vi "Select Trans.vi"(8 "error in (no error)":errorcluster) -> (0 "error out":errorcluster, 3 "Amplifier Type 2":T1)   [LabVIEW 2015]
uses:
  controls/OpAmp Amplifiers.ctl
  controls/AmplifierTypes.ctl
panel:
  in  "Cancel Button":bool
  in  "Amplifier Type":T1 caption="Trans Type"
  in  "Opamp Type":T2 caption="OpAmp"
  in  "EC":bool
  in  "CC":bool
  in  "BC":bool
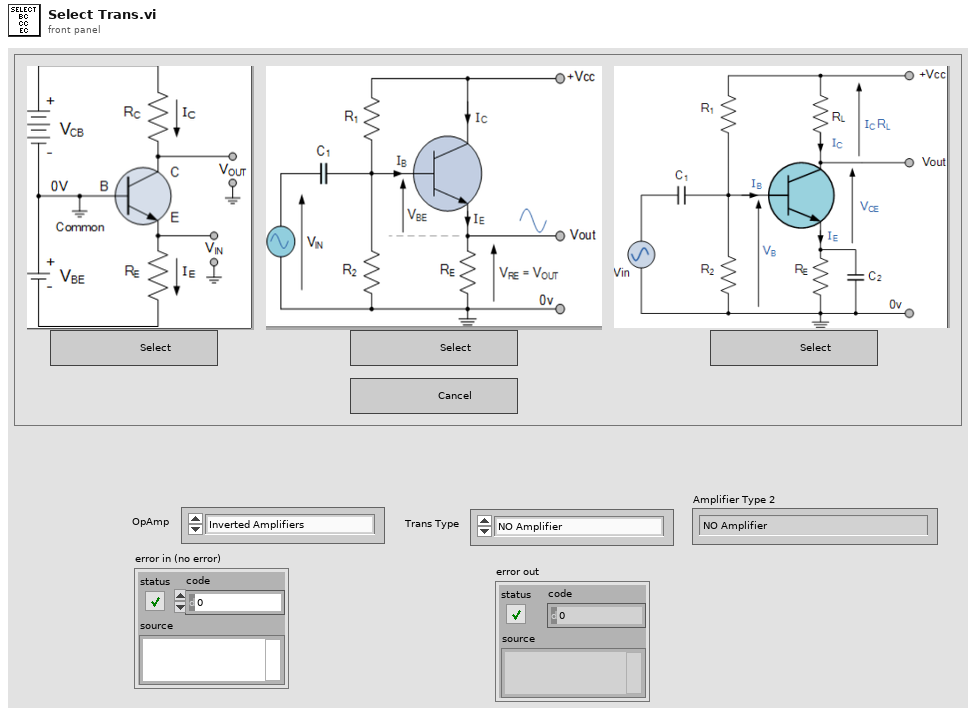
[diagram p1: front panel]
types:
  T1 = typedef "AmplifierTypes.ctl" = enum8{"NO Amplifier", "EC", "BC", "CC"}
  T2 = typedef "OpAmp Amplifiers.ctl" = enum8{"Inverted Amplifiers", "non-Inverted Amplifiers", "NO Amplifier"}
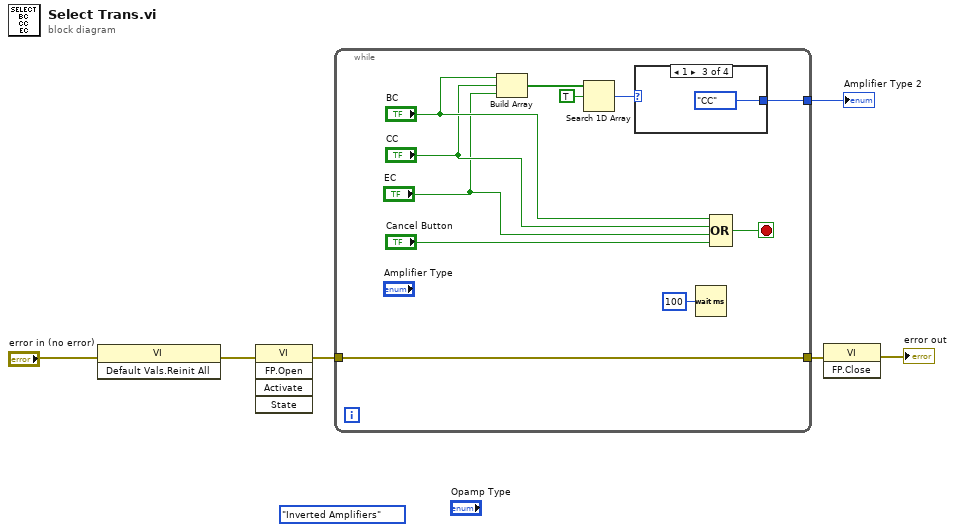
[diagram p0: block diagram]
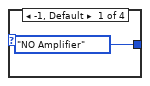
[diagram p2: hidden frame]
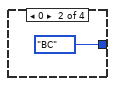
[diagram p3: hidden frame]
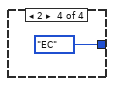
[diagram p4: hidden frame]
diagram:
  (unwired) OpAmp_Amplifiers."Inverted Amplifiers" ("Opamp Type")
  n1 = invoke class="VI" method="Default Vals.Reinit All"(error in="error in (no error)") -> (error out=w3:errorcluster)  [unwired: 2 in, 2 out]
  n2 = invoke class="VI" method="FP.Open"(error in=w3) -> (error out=w5:errorcluster)  [unwired: 4 in, 4 out]
  n3 = while {
    tunnel: [w9] -> w6
    tunnel: w5 -> [w8]
    tunnel: [w8] -> w1
    stop <- w17 stop-if-true
    n4 = Build Array("BC", "CC", "EC") -> (w12:bool[])
    n5 = Search 1D Array(1D array=w12, element=TRUE) -> (index of element=w10:i32)  [unwired: 1 in]
    n6 = case shown="1" w10 {
      tunnel: [AmplifierTypes."NO Amplifier" ("Amplifier Type") AmplifierTypes."BC" ("Amplifier Type") AmplifierTypes."CC" ("Amplifier Type") AmplifierTypes."EC" ("Amplifier Type")] -> w9
      frame -1, Default {
      }
      frame 0 {
      }
      frame 1 {
      }
      frame 2 {
      }
    }
    n7 = Wait (ms)(milliseconds to wait=u32 100) -> ()  [unwired: 1 out]
    n8 = Compound Arithmetic op=OR("BC", "CC", "EC", "Cancel Button") -> (w17:bool)
  }
  "Amplifier Type 2" <- w6
  n9 = invoke class="VI" method="FP.Close"(error in=w1) -> (error out=→"error out":errorcluster)  [unwired: 2 in, 2 out]
